vi "cv_07_07.vi"() -> ()   [LabVIEW 2013]
panel:
  out "Array 2":dbl[](array[numeric])
  in  "Array":dbl[](array[numeric])
  in  "Numeric":dbl
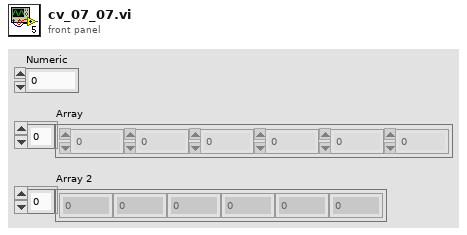
[diagram p1: front panel]
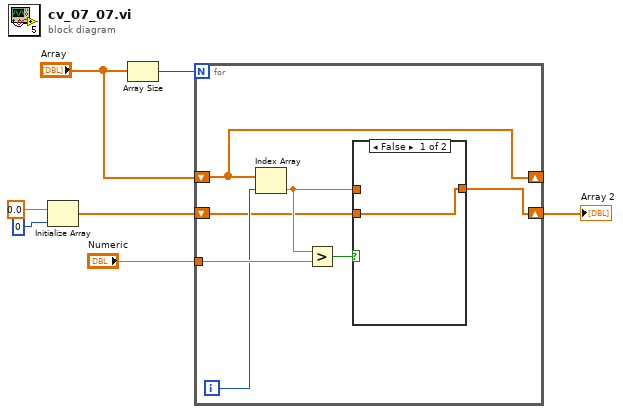
[diagram p0: block diagram]
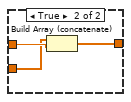
[diagram p2: hidden frame]
diagram:
  n1 = Initialize Array(0.0, 0) -> (w3:dbl[])
  n2 = Array Size(array="Array") -> (size(s)=w7:i32)
  n3 = for {
    N: w7 -> [_]
    shift-right: [w14] -> _
    shift-left: "Array" -> [w14]
    shift-right: [w8] -> w2
    shift-left: w3 -> [w9]
    tunnel: "Numeric" -> [w13]
    i -> [w12]
    n4 = Index Array(array=w14, index=w12) -> (element=w10:dbl)
    n5 = Greater?(x=w10, y=w13) -> (0:w11:bool)
    n6 = case shown="False" w11 {
      tunnel: w10 -> [_ w18]
      tunnel: w9 -> [w15 w17]
      tunnel: [w15 w16] -> w8
      frame False {
      }
      frame True {
        n7 = Build Array (concatenate)(w17, w18) -> (w16:dbl[])
      }
    }
  }
  "Array 2" <- w2
